vi "Function_runNstop.vi"(5 "VISA resource name in":refnum<visa-resource-name>, 7 "error in":errorcluster, 10 "condition":i32 caption="comdition", 11 "Server addr":string) -> (4 "VISA resource name out":refnum<visa-resource-name>, 6 "error out":errorcluster)   [LabVIEW 2020]
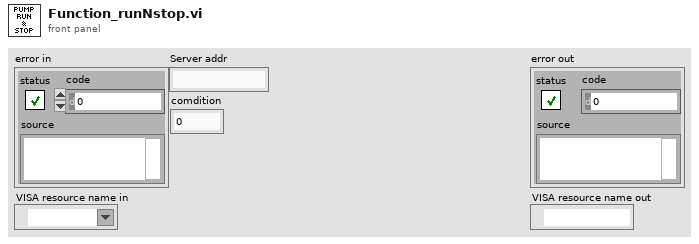
[diagram p1: front panel]
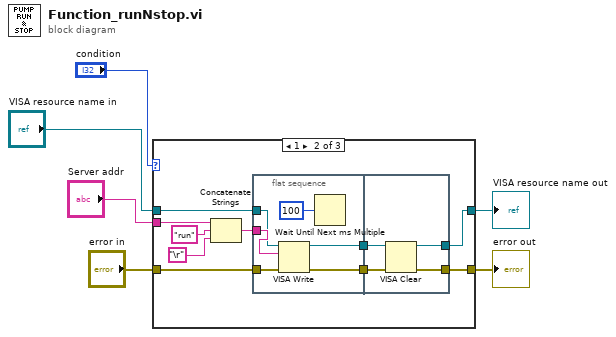
[diagram p0: block diagram]
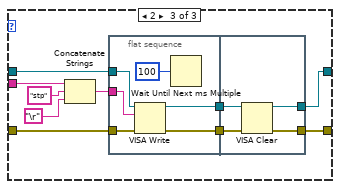
[diagram p3: hidden frame]
diagram:
  n1 = case shown="1" "condition" {
    tunnel: [w8 w11 w35] -> w6
    tunnel: [w7 w10 w34] -> w5
    tunnel: "VISA resource name in" -> [w8 w15 w33]
    tunnel: "error in" -> [w7 w14 w32]
    tunnel: "Server addr" -> [_ w9 w29]
    frame 0, Default {
    }
    frame 1 {
      n2 = Concatenate Strings(w9, "run" ("string"), "\r") -> (w16:string)
      n3 = flat-sequence {
        tunnel: w16 -> [w24]
        tunnel: w15 -> [w23]
        tunnel: w14 -> [w22]
        tunnel: [w21] -> w13
        tunnel: [w20] -> w12
        tunnel: w13 -> [w28]
        tunnel: w12 -> [w27]
        tunnel: [w26] -> w11
        tunnel: [w25] -> w10
        frame #0 {
          n4 = VISA Write(VISA resource name=w23, write buffer=w24, error in (no error)=w22) -> (VISA resource name out=w21:refnum<visa-resource-name>, error out=w20:errorcluster)  [unwired: 1 out]
          n5 = Wait Until Next ms Multiple(millisecond multiple=u32 100) -> ()  [unwired: 1 out]
        }
        frame #1 {
          n6 = VISA Clear(VISA resource name=w28, error in (no error)=w27) -> (VISA resource name out=w26:refnum<visa-resource-name>, error out=w25:errorcluster)
        }
      }
    }
    frame 2 {
      n7 = Concatenate Strings(w29, "stp" ("string"), "\r") -> (w36:string)
      n8 = flat-sequence {
        tunnel: w36 -> [w44]
        tunnel: w33 -> [w41]
        tunnel: w32 -> [w40]
        tunnel: [w43] -> w31
        tunnel: [w42] -> w30
        tunnel: [w48] -> w34
        tunnel: [w45] -> w35
        tunnel: w31 -> [w47]
        tunnel: w30 -> [w46]
        frame #0 {
          n9 = VISA Write(VISA resource name=w41, write buffer=w44, error in (no error)=w40) -> (VISA resource name out=w43:refnum<visa-resource-name>, error out=w42:errorcluster)  [unwired: 1 out]
          n10 = Wait Until Next ms Multiple(millisecond multiple=u32 100) -> ()  [unwired: 1 out]
        }
        frame #1 {
          n11 = VISA Clear(VISA resource name=w47, error in (no error)=w46) -> (VISA resource name out=w45:refnum<visa-resource-name>, error out=w48:errorcluster)
        }
      }
    }
  }
  "error out" <- w5
  "VISA resource name out" <- w6
